vi "wsConnection_random_number.vi"() -> ()   [LabVIEW 2013]
uses:
  <vilib>/MediaMongrels Ltd/WebSockets/WebSockets/WebSockets.lvlib
panel:
  in  "Frequency":dbl
  out "Number":dbl
  in  "stop":bool
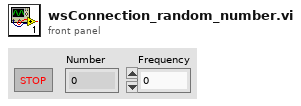
[diagram p1: front panel]
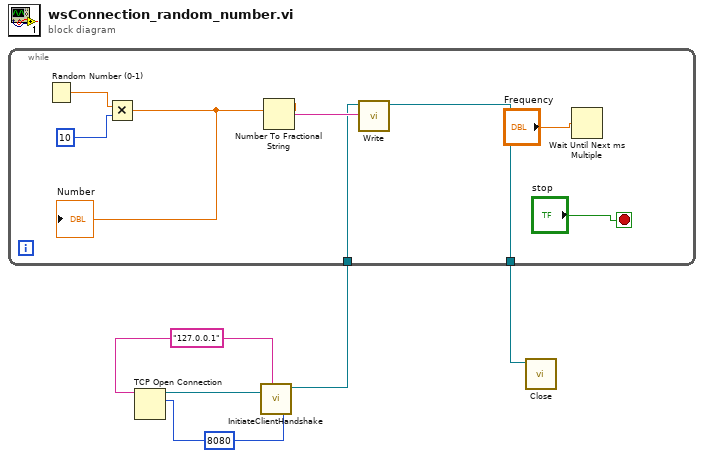
[diagram p0: block diagram]
diagram:
  w4 = "127.0.0.1"
  w5 = 8080
  n1 = TCP Open Connection(address=w4, remote port or service name=w5) -> (connection ID=w3:refnum<k5>)  [unwired: 3 in, 1 out]
  n2 = call <vilib>:"InitiateClientHandshake.vi"("remote port or service name"=w5, "address"=w4, "WebSocket Connection in"=w3) -> ("WebSocket Connection out"=w2:refnum<k5>)  [unwired: 6 in, 2 out]
  n3 = while {
    tunnel: [w7] -> w1
    tunnel: w2 -> [w6]
    stop <- "stop" stop-if-true
    n4 = Random Number (0-1)() -> (number: 0 to 1=w12:dbl)
    n5 = Multiply(x=w12, y=10) -> (x*y=w9:dbl)
    "Number" <- w9
    n6 = Number To Fractional String(number=w9) -> (F-format string=w10:string)  [unwired: 3 in]
    n7 = call <vilib>:"Write.vi"("Data"=w10, "WebSocket Connection in"=w6) -> ("WebSocket Connection out"=w7:refnum<k5>)  [unwired: 8 in, 1 out]
    n8 = Wait Until Next ms Multiple(millisecond multiple="Frequency") -> ()  [unwired: 1 out]
  }
  n9 = call <vilib>:"Close.vi"("WebSocket Connection in"=w1) -> ()  [unwired: 9 in, 2 out]
